vi "safe_data.vi"(2 "record(s)":dbl[][](array[numeric]), 3 "default name":string="TEMP.DAT") -> ()   [LabVIEW 2011]
panel:
  in  "start path":path=path "X:/Dropbox/UoA/Cool Amps/Labview/meas_data"
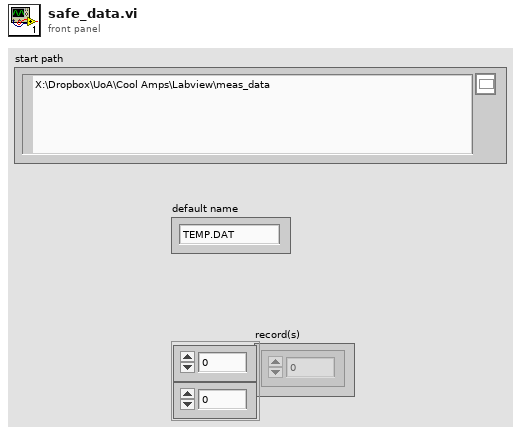
[diagram p1: front panel]
types:
  T1 = enum16{"open", "replace", "create", "open or create", "replace or create", "replace or create with confirmation"}
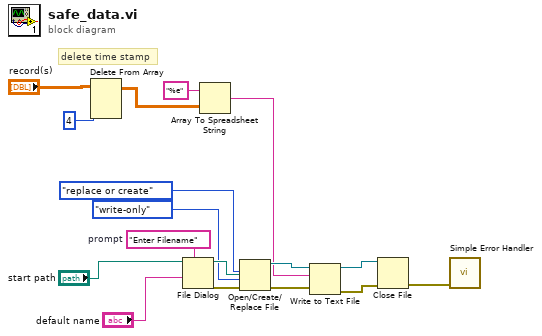
[diagram p0: block diagram]
diagram:
  w17 = "Enter Filename"  # prompt
  # "delete time stamp"
  n1 = Delete From Array(array="record(s)", index (col)=4 ("index (row)")) -> (array with subset deleted=w3:dbl[][])  [unwired: 2 in, 1 out]
  n2 = File Dialog(7:w17, 9:"default name", 11:"start path") -> (0:w12:errorcluster, 3:w13:path)  [unwired: 4 in, 2 out]
  n3 = Array To Spreadsheet String(array=w3, 3:"%e") -> (spreadsheet string=w5:string)  [unwired: 1 in]
  n4 = Open/Create/Replace File(file path (use dialog)=w13, error in=w12, operation (0:open)=T1."replace or create", access (0:read/write)=enum16{"read/write", "read-only", "write-only"}."write-only") -> (refnum out=w9:refnum<file>, error out=w8:errorcluster)  [unwired: 2 in, 1 out]
  n5 = Write to Text File(file (use dialog)=w9, text=w5, error in=w8) -> (refnum out=w7:refnum<file>, error out=w6:errorcluster)  [unwired: 1 in, 1 out]
  n6 = Close File(refnum=w7, error in=w6) -> (error out=w16:errorcluster)  [unwired: 1 out]
  n7 = call <vilib>:"Simple Error Handler.vi"("error in (no error)"=w16) -> ()  [unwired: 4 in, 5 out]
